vi "Open.vi"(8 "Error In":errorcluster, 9 "Number of LEDs":u16, 10 "Data Channel":u8, 11 "LINX Resource":T1={"IO"=enum."Remote", "Interface"=enum."Serial", "LINX Device Config"={"Interface"=enum."Serial", "COM Port"="COM13", "TCP Configuration"={"IP Address"="", "Port"=0}, "Device Family"=1, "Device ID"=1, "Device Name"="myRIO-1900", "TCP Ref"=refnum, "Channels"={"DI"=[0, 1, 2, 3, 4, 5, 6, 7, 8, 9, 10, 11, 12, 13, 14, 15, 16, 17, 18, 19, 20, 21, 22, 23, 24, 25, 26, 27, 28, 29, 30, 31, 32, 33, 34, 35, 36, 37, 38, 39, 40, 41, 42, 43, 44, 45, 46], "DO"=[0, 1, 2, 3, 4, 5, 6, 7, 8, 9, 10, 11, 12, 13, 14, 15, 16, 17, 18, 19, 20, 21, 22, 23, 24, 25, 26, 27, 28, 29, 30, 31, 32, 33, 34, 35, 36, 37, 38, 39, 40, 41, 42, 43, 44, 45, 46], "AI"=[0, 1, 2, 3, 4, 5, 6, 7, 8, 9, 10, 11], "AO"=[], "PWM"=[3, 5, 6, 9, 10], "QE"=[], "UART"=[0, 1], "I2C 2"=[0], "SPI"=[0], "CAN"=[], "Servo"=[], "AI Ref (V)"=0.0, "AI Resolution (Bits)"=0, "AO Ref (V)"=0.0, "AO Resolution (Bits)"=0}}}) -> (0 "Error Out":errorcluster={"status"=FALSE, "code"=1073676294, "source"="VISA Read in LVH-LINX.lvlib:Device.lvlib:Serial Read.vi->LVH-LINX.lvlib:Device.lvlib:Wait For Packet.vi->LVH-LINX.lvlib:Device.lvlib:Send Command.vi->LVH-LINX.lvlib:Device.lvlib:Get DIO Channels.vi->LVH-LINX.lvlib:Device.lvlib:Load Device Config.vi->LVH-LINX.lvlib:Device.lvlib:Initialize Device.vi->LVH-LINX.lvlib:Initialize.vi->Untitled 2"}, 3 "LINX Resource":T1={"IO"=enum."Remote", "Interface"=enum."Serial", "LINX Device Config"={"Interface"=enum."Serial", "COM Port"="COM13", "TCP Configuration"={"IP Address"="", "Port"=0}, "Device Family"=1, "Device ID"=1, "Device Name"="myRIO-1900", "TCP Ref"=refnum, "Channels"={"DI"=[0, 1, 2, 3, 4, 5, 6, 7, 8, 9, 10, 11, 12, 13, 14, 15, 16, 17, 18, 19, 20, 21, 22, 23, 24, 25, 26, 27, 28, 29, 30, 31, 32, 33, 34, 35, 36, 37, 38, 39, 40, 41, 42, 43, 44, 45, 46], "DO"=[0, 1, 2, 3, 4, 5, 6, 7, 8, 9, 10, 11, 12, 13, 14, 15, 16, 17, 18, 19, 20, 21, 22, 23, 24, 25, 26, 27, 28, 29, 30, 31, 32, 33, 34, 35, 36, 37, 38, 39, 40, 41, 42, 43, 44, 45, 46], "AI"=[0, 1, 2, 3, 4, 5, 6, 7, 8, 9, 10, 11], "AO"=[], "PWM"=[3, 5, 6, 9, 10], "QE"=[], "UART"=[0, 1], "I2C 2"=[0], "SPI"=[0], "CAN"=[], "Servo"=[], "AI Ref (V)"=0.0, "AI Resolution (Bits)"=0, "AO Ref (V)"=0.0, "AO Resolution (Bits)"=0}}})   [LabVIEW 2020, in "LMH-LINX.lvlib" / "WS2812.lvlib"]
doc: "Open the WS2812 controller. This function will allocate memory on the device to store the RGB data. If the device is unable to allocate memory an error is returned.\n\nNote: WS2812 Functions Are Currently Only Supported on chipKIT WF32 and Max32.\n\nWF32 must use pin 11 as the data channel\nMax32 must use pin 43 if jumper JP4 is set to slave and 51 if JP4 is set to master."
uses:
  WS2812.lvlib
  Private/Type Defs/LINX Ref.ctl
  Private/Type Defs/Platform.ctl
  Private/Type Defs/Interface.ctl
  Private/Device/Type Defs/LINX Device Config.ctl
  Private/Device/Type Defs/TCP Config.ctl
  Private/Device/Type Defs/Channels.ctl
  Private/Type Defs/Error Type.ctl
  Private/Device/Device.lvlib
  LMH-LINX.lvlib
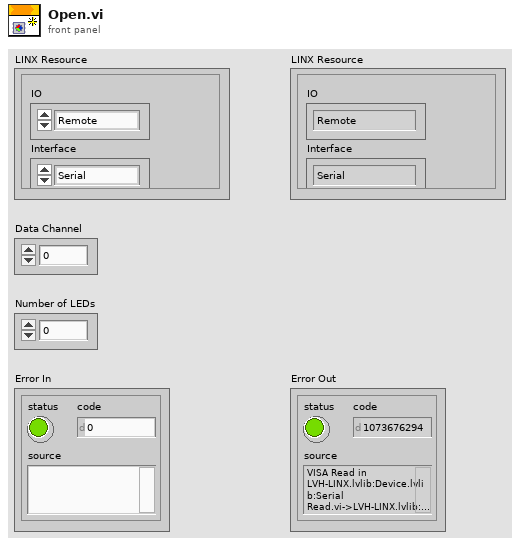
[diagram p1: front panel]
types:
  T1 = typedef "LMH-LINX.lvlib/LINX Ref.ctl" = cluster{"IO":T2, "Interface":T3, "LINX Device Config":T4}
  T2 = typedef "LMH-LINX.lvlib/Platform.ctl" = enum16{"Remote", "Local"}
  T3 = typedef "LMH-LINX.lvlib/Interface.ctl" = enum16{"Serial", "TCP"}
  T4 = typedef "Device.lvlib/LINX Device Config.ctl" = cluster{"Interface":T3, "COM Port":refnum<visa-resource-name>, "TCP Configuration":T5, "Device Family":u8, "Device ID":u8, "Device Name":string, "TCP Ref":refnum<k5>, "Channels":T6}
  T5 = typedef "Device.lvlib/TCP Config.ctl" = cluster{"IP Address":string, "Port":u16}
  T6 = typedef "LMH-LINX.lvlib/Channels.ctl" = cluster{"DI":u8[], "DO":u8[], "AI":u8[], "AO":u8[], "PWM":u8[], "QE":u8[], "UART":u8[], "I2C 2":u8[], "SPI":u8[], "CAN":u8[], "Servo":u8[], "AI Ref (V)":dbl, "AI Resolution (Bits)":u8, "AO Ref (V)":dbl, "AO Resolution (Bits)":u8}
  T7 = typedef "LMH-LINX.lvlib/Error Type.ctl" = enum16{"Unknown", "Timeout", "Corrupt Return Packet", "Unable To Connect", "Command Not Supported", "Channel DNE", "Invalid COM Config", "Firmware Version Mismatch", "myRIO Support", "CMD Specific Error", "Local IO Not Supported"}
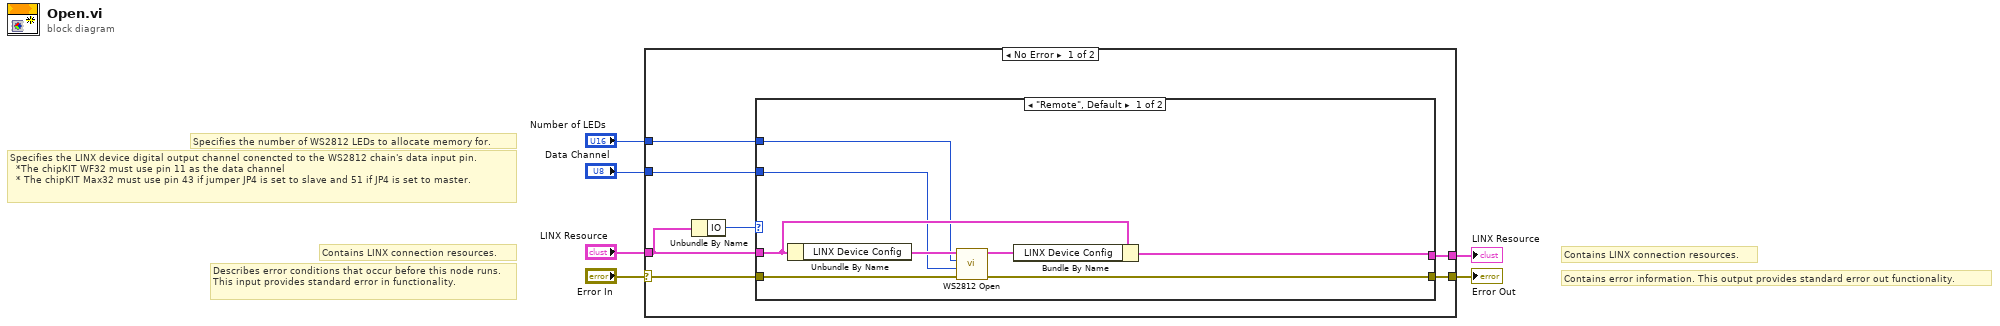
[diagram p0: block diagram]
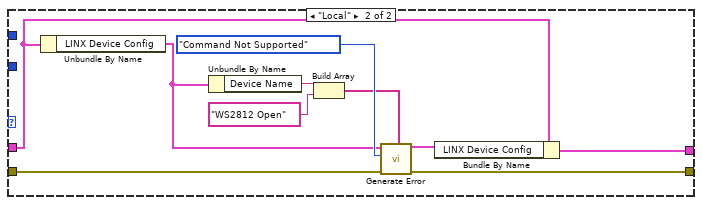
[diagram p2: hidden frame]
diagram:
  # "Specifies the LINX device digital output channel conencted to the WS2812 chain's data input pin. \n  *The chipKIT WF32 must use pin 11 as the data channel\n  * The chipKIT Max32 must use pin 43 if jumper JP4 is set to slave and 51 if JP4 is set to master."
  # "Specifies the number of WS2812 LEDs to allocate memory for."
  # "Contains LINX connection resources."
  # "Contains error information. This output provides standard error out functionality."
  # "Contains LINX connection resources."
  # "Describes error conditions that occur before this node runs. This input provides standard error in functionality."
  n1 = case shown="No Error" "Error In" {
    selector: "Error In" -> [w12 w32]
    tunnel: "LINX Resource" -> [w11 w33]
    tunnel: [w10 w32] -> w4
    tunnel: [w9 w33] -> w3
    tunnel: "Data Channel" -> [w8 _]
    tunnel: "Number of LEDs" -> [w7 _]
    frame No Error {
      n2 = Unbundle By Name(w11) -> ("IO"=w13:T2)
      n3 = case shown="\"Remote\", Default" w13 {
        tunnel: w12 -> [w21 w25]
        tunnel: w11 -> [w18 w22]
        tunnel: [w17 w24] -> w10
        tunnel: [w16 w23] -> w9
        tunnel: w8 -> [w15 _]
        tunnel: w7 -> [w14 _]
        frame "Remote", Default {
          n4 = Unbundle By Name(w18) -> ("LINX Device Config"=w20:T4)
          n5 = call "WS2812 Open.vi"("Error In"=w21, "Data Channel"=w15, "Number of LEDs"=w14, "LINX Device Config"=w20) -> ("Error Out"=w17:errorcluster, "LINX Device Config"=w19:T4)  [unwired: 6 in]
          n6 = Bundle By Name(cluster=w18, "LINX Device Config"=w19) -> (w16:T1)
        }
        frame "Local" {
          n7 = Unbundle By Name(w22) -> ("LINX Device Config"=w27:T4)
          n8 = Unbundle By Name(w27) -> ("Device Name"=w31:string)
          n9 = Build Array(w31, "WS2812 Open") -> (w28:string[])
          n10 = call "Generate Error.vi"("Error In"=w25, "Arguments"=w28, "Error Type"=Error_Type."Command Not Supported", "LINX Device Config"=w27) -> ("Error Out"=w24:errorcluster, "Dup LINX Device Config"=w26:T4)  [unwired: 6 in]
          n11 = Bundle By Name(cluster=w22, "LINX Device Config"=w26) -> (w23:T1)
        }
      }
    }
    frame Error {
    }
  }
  "Error Out" <- w4
  "LINX Resource" <- w3
